vi "Servo Pulse Gen..vi"() -> ()   [LabVIEW 2020]
uses:
  Slide Servo.ctl
  Galobal variable_TI.vi
  Project Setup/Globle Variable/GR_Servo.vi
panel:
  out "Enum":T1
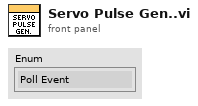
[diagram p1: front panel]
types:
  T1 = typedef "Slide Servo.ctl" = enum16{"Poll Event", "Servo CMD", "Slide Servo Home ", "Exit"}
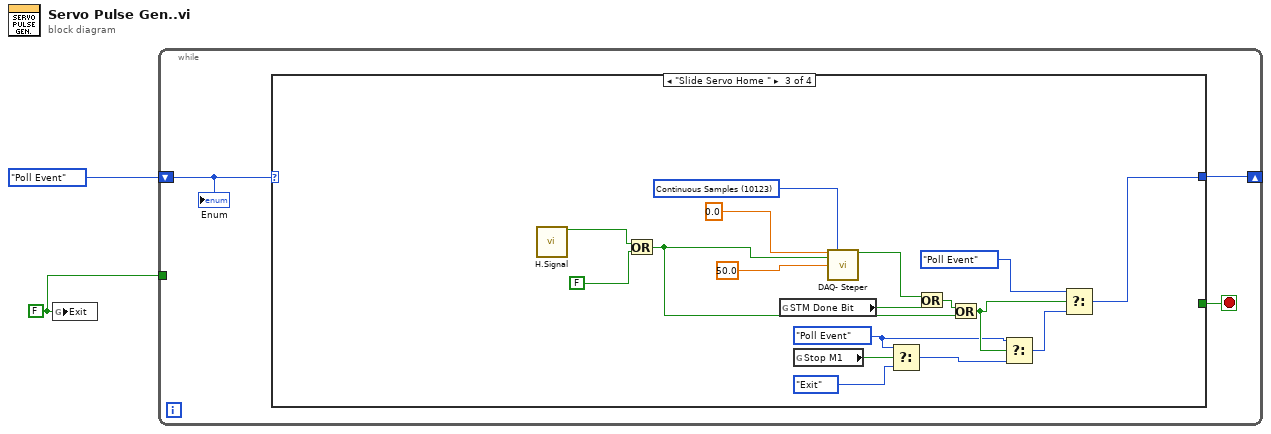
[diagram p0: block diagram]
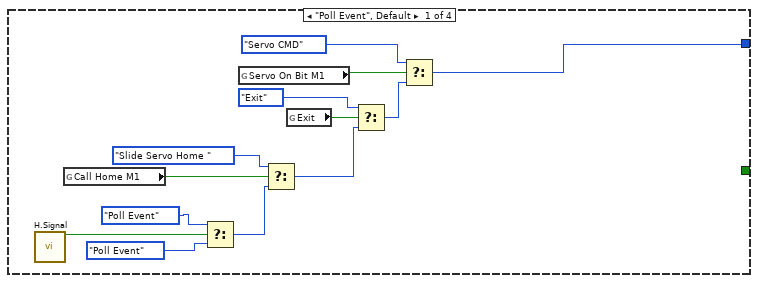
[diagram p2: hidden frame]
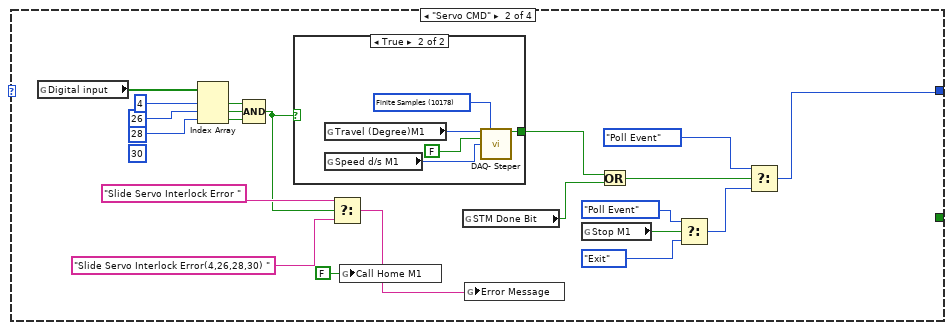
[diagram p3: hidden frame]
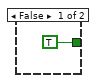
[diagram p4: hidden frame]
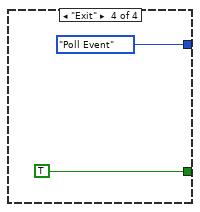
[diagram p5: hidden frame]
diagram:
  w1 = FALSE ("Exit")
  n1 = global write "Galobal variable_TI.vi" "Exit"(w1) -> ()
  n2 = while {
    shift-right: [w4] -> _
    shift-left: Slide_Servo."Poll Event" ("Enum") -> [w5]
    tunnel: w1 -> [_]
    stop <- w3 stop-if-true
    n3 = case shown="\"Slide Servo Home \"" w5 {
      tunnel: [w13 w35 w49 Slide_Servo."Poll Event" ("Enum")] -> w4
      tunnel: [_ _ _ TRUE] -> w3
      frame "Poll Event", Default {
        n4 = call "H.Signal.vi"() -> ("Slide servo home RS"=w9:bool)  [unwired: 10 in, 5 out]
        n5 = global read "Galobal variable_TI.vi" "Call Home M1"() -> (w11:bool)
        n6 = Select(t=Slide_Servo."Poll Event" ("Enum"), s=w9, f=Slide_Servo."Poll Event" ("Enum")) -> (s? t:f=w7:T1)
        n7 = global read "GR_Servo.vi" "Servo On Bit M1"() -> (w16:bool)
        n8 = Select(t=Slide_Servo."Slide Servo Home " ("Enum"), s=w11, f=w7) -> (s? t:f=w10:T1)
        n9 = global read "Galobal variable_TI.vi" "Exit"() -> (w17:bool)
        n10 = Select(t=Slide_Servo."Exit" ("Enum"), s=w17, f=w10) -> (s? t:f=w18:T1)
        n11 = Select(t=Slide_Servo."Servo CMD" ("Enum"), s=w16, f=w18) -> (s? t:f=w13:T1)
      }
      frame "Servo CMD" {
        (unwired) 30 ("index")
        n12 = global read "Galobal variable_TI.vi" "Digital input"() -> (w29:bool[])
        n13 = Index Array(array=w29, index #1=4 ("index"), index #2=26 ("index"), index #3=28 ("index")) -> (element #1=w23:bool, element #2=w25:bool, element #3=w24:bool)
        n14 = Compound Arithmetic op=AND(w23, w25, w24) -> (w19:bool)
        n15 = case shown="True" w19 {
          tunnel: [TRUE ("Task Done Bit") w43] -> w39
          frame False {
          }
          frame True {
            w41 = 10178 items=["Finite Samples"=10178, "Continuous Samples"=10123, "Hardware Timed Single Point"=12522] ("Mode")
            n16 = global read "GR_Servo.vi" "Travel (Degree)M1"() -> (w44:i32)
            n17 = global read "GR_Servo.vi" "Speed d/s M1"() -> (w45:i32)
            n18 = call "DAQ- Steper.vi"("Travel (Degree)"=w44, "Mode"=w41, "Home Condition"=FALSE, "Speed d/s"=w45) -> ("Task Done Bit"=w43:bool)  [unwired: 10 in, 1 out]
          }
        }
        n19 = Select(t="Slide Servo Interlock Error ", s=w19, f="Slide Servo Interlock Error(4,26,28,30) ") -> (s? t:f=w20:string)
        n20 = global write "Galobal variable_TI.vi" "Call Home M1"(FALSE ("Call Home M1")) -> ()
        n21 = global read "Galobal variable_TI.vi" "STM Done Bit"() -> (w38:bool)
        n22 = global write "GR_Servo.vi" "Error Message"(w20) -> ()
        n23 = global read "Galobal variable_TI.vi" "Stop M1"() -> (w34:bool)
        n24 = Or(x=w39, y=w38) -> (x .or. y?=w37:bool)
        n25 = Select(t=Slide_Servo."Poll Event" ("Enum"), s=w34, f=Slide_Servo."Exit" ("Enum")) -> (s? t:f=w31:T1)
        n26 = Select(t=Slide_Servo."Poll Event" ("Enum"), s=w37, f=w31) -> (s? t:f=w35:T1)
      }
      frame "Slide Servo Home " {
        w48 = 10123 items=["Finite Samples"=10178, "Continuous Samples"=10123, "Hardware Timed Single Point"=12522] ("Mode")
        w51 = Slide_Servo."Poll Event" ("Enum")
        n27 = call "H.Signal.vi"() -> ("Slide servo home RS"=w62:bool)  [unwired: 10 in, 5 out]
        n28 = Or(x=w62, y=FALSE) -> (x .or. y?=w56:bool)
        n29 = global read "Galobal variable_TI.vi" "STM Done Bit"() -> (w60:bool)
        n30 = global read "Galobal variable_TI.vi" "Stop M1"() -> (w55:bool)
        n31 = call "DAQ- Steper.vi"("Travel (Degree)"=0.0, "Mode"=w48, "Home Condition"=w56, "Speed d/s"=50.0) -> ("Task Done Bit"=w61:bool)  [unwired: 10 in, 1 out]
        n32 = Select(t=w51, s=w55, f=Slide_Servo."Exit" ("Enum")) -> (s? t:f=w52:T1)
        n33 = Or(x=w61, y=w60) -> (x .or. y?=w57:bool)
        n34 = Or(x=w57, y=w56) -> (x .or. y?=w53:bool)
        n35 = Select(t=w51, s=w53, f=w52) -> (s? t:f=w50:T1)
        n36 = Select(t=Slide_Servo."Poll Event" ("Enum"), s=w53, f=w50) -> (s? t:f=w49:T1)
      }
      frame "Exit" {
      }
    }
    "Enum" <- w5
  }
